vi "Resistance Test_ver2_2.vi"(0 "DMM ref in":refnum<visa-resource-name>, 1 "Measure\nMax Voltage":dbl=100.0, 2 "Resistance Test REF":refnum<vi>, 3 "Resistance Test Stop REF":refnum<vi>, 5 "DMM error in":errorcluster, 7 "Channel  Count":i32, 9 "ESP32 ref in":refnum<visa-resource-name>="COM4", 11 "ESP32 error in":errorcluster, 12 "Wait Current Stable Period":u32, 13 "Manual Trigger Delay (1 s)":dbl=1.0, 14 "Current Sense \nResitance Array":dbl[](array[numeric])) -> (10 "ESP32 ref out":refnum<visa-resource-name>, 15 "ESP32 error out":errorcluster)   [LabVIEW 2023]
uses:
  <instrlib>/Agilent 3446X Series/Agilent 3446X Series.lvlib
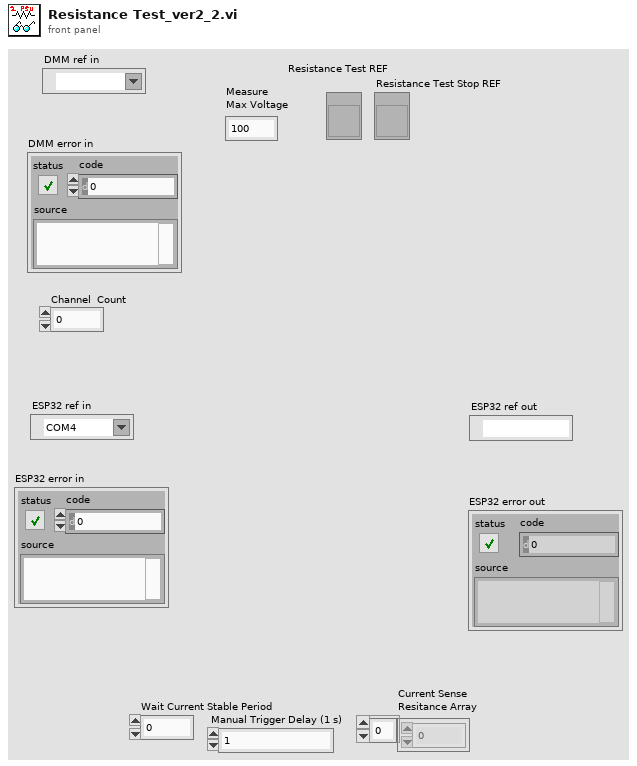
[diagram p1: front panel]
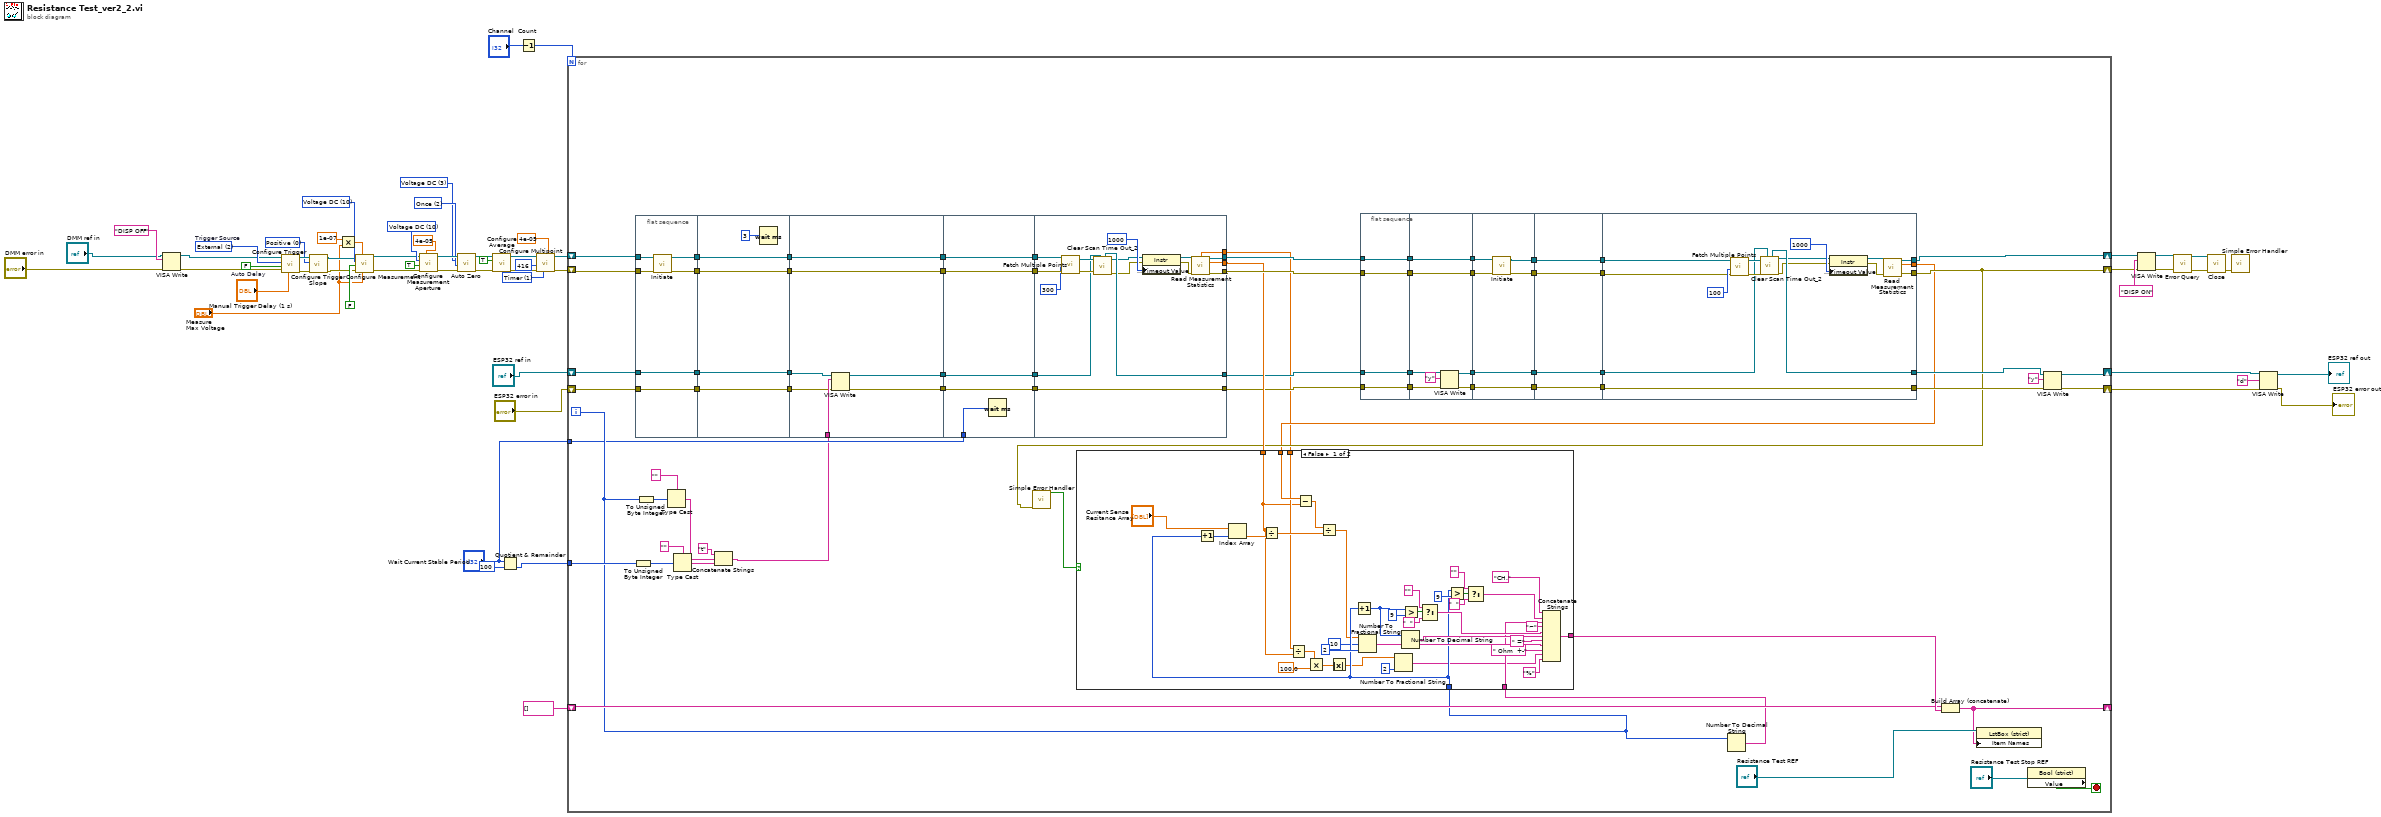
[diagram p0: block diagram]
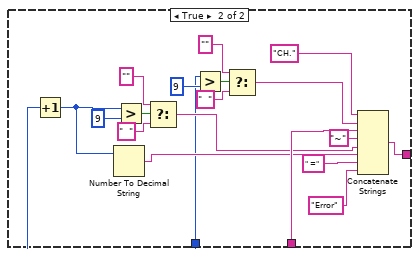
[diagram p2: hidden frame]
diagram:
  w19 = 0 items=["Positive", "Negative"] ("Trigger Edge (1: Negative)")
  w17 = 2 items=["Immediate", "Software (Bus)", "External"]  # Trigger Source
  w18 = FALSE  # Auto Delay
  w25 = 10 items=["Continuity", "Current AC", "Current DC", "Diode", "Frequency", "Resistance 4-wire", "Period", "Resistance 2-wire", "Temperature", "Voltage AC", "Voltage DC", "Voltage DC Ratio", "Capacitance"] ("Measurement Function (10: Voltage DC)")
  w29 = 1 items=["Immediate", "Timer"] ("Sample Source (0: Immediate)")
  w36 = 3 items=["Current DC", "Resistance", "Temperature", "Voltage DC"] ("Zero Type (0: Current DC)")
  w37 = 2 items=["Disable", "Enable", "Once"] ("Auto Zero (1: Enable)")
  w33 = 10 items=["Continuity", "Current AC", "Current DC", "Diode", "Frequency", "Resistance 4-wire", "Period", "Resistance 2-wire", "Temperature", "Voltage AC", "Voltage DC", "Voltage DC Ratio", "Capacitance"] ("Measurement Function (0: Continuity)")
  n1 = VISA Write(VISA resource name="DMM ref in", write buffer="DISP OFF", error in (no error)="DMM error in") -> (VISA resource name out=w4:refnum<visa-resource-name>, error out=w3:errorcluster)  [unwired: 1 out]
  n2 = call <instrlib>:"Configure Trigger.vi"("Manual Trigger Delay (1 s)"="Manual Trigger Delay (1 s)", "error in (no error)"=w3, "Auto Delay (F:Disable)"=w18, "Trigger Source (0: Immediate)"=w17, "VISA resource name"=w4) -> ("error out"=w21:errorcluster, "VISA resource name out"=w20:refnum<visa-resource-name>)  [unwired: 1 in, 4 out]
  n3 = call <instrlib>:"Configure Trigger Slope.vi"("error in (no error)"=w21, "Trigger Edge (1: Negative)"=w19, "VISA resource name"=w20) -> ("error out"=w15:errorcluster, "VISA resource name out"=w16:refnum<visa-resource-name>)  [unwired: 7 in]
  n4 = Multiply(x=1e-07, y="Measure\nMax Voltage") -> (x*y=w26:dbl)
  n5 = call <instrlib>:"Configure Measurement.vi"("Manual Range (1)"="Measure\nMax Voltage", "Absolute Resolution (1E-6)"=w26, "error in (no error)"=w15, "Auto Range (T: Enable)"=FALSE, "Measurement Function (10: Voltage DC)"=w25, "VISA resource name"=w16) -> ("error out"=w22:errorcluster, "VISA resource name out"=w23:refnum<visa-resource-name>)  [unwired: 4 out]
  n6 = call <instrlib>:"Configure Measurement Aperture.vi"("Aperture Time (0.1s)"=4e-05, "error in (no error)"=w22, "Enable Aperture (F: Disable)"=TRUE, "Measurement Function (0: Continuity)"=w33, "VISA resource name"=w23) -> ("error out"=w40:errorcluster, "VISA resource name out"=w39:refnum<visa-resource-name>)  [unwired: 5 in]
  n7 = call <instrlib>:"Auto Zero.vi"("error in (no error)"=w40, "Auto Zero (1: Enable)"=w37, "Zero Type (0: Current DC)"=w36, "VISA resource name"=w39) -> ("error out"=w42:errorcluster, "VISA resource name out"=w41:refnum<visa-resource-name>)  [unwired: 6 in]
  n8 = call <instrlib>:"Configure Average.vi"("error in (no error)"=w42, "Enable Statistics (F: Disable)"=TRUE, "VISA resource name"=w41) -> ("error out"=w31:errorcluster, "VISA resource name out"=w32:refnum<visa-resource-name>)  [unwired: 7 in]
  n9 = Quotient & Remainder(x="Wait Current Stable Period", y=100) -> (floor(x/y)=w11:u32)  [unwired: 1 out]
  n10 = Decrement(x="Channel  Count") -> (x-1=w9:i32)
  n11 = call <instrlib>:"Configure Multipoint.vi"("Sample Interval (1 Second)"=4e-05, "Sample Source (0: Immediate)"=w29, "error in (no error)"=w31, "Sample Count (1)"=416, "VISA resource name"=w32) -> ("error out"=w13:errorcluster, "VISA resource name out"=w14:refnum<visa-resource-name>)  [unwired: 2 in, 3 out]
  n12 = for {
    N: w9 -> [_]
    shift-right: [w82] -> w44
    shift-left: "ESP32 ref in" -> [w111]
    shift-right: [w80] -> w10
    shift-left: "ESP32 error in" -> [w109]
    shift-right: [w78] -> w45
    shift-left: w13 -> [w115]
    shift-right: [w121] -> w46
    shift-left: w14 -> [w116]
    shift-right: [w122] -> _
    shift-left: string[] [] -> [w124]
    tunnel: w11 -> [w99]
    tunnel: "Wait Current Stable Period" -> [w86]
    i -> [w97]
    stop <- w126 stop-if-true
    n13 = To Unsigned Byte Integer(number=w99) -> (unsigned 8bit integer=w103:u8)
    n14 = flat-sequence {
      tunnel: w115 -> [w225]
      tunnel: w116 -> [w227]
      tunnel: [w226] -> w120
      tunnel: [w224] -> w119
      tunnel: [w223] -> w112
      tunnel: w111 -> [w223]
      tunnel: w109 -> [w222]
      tunnel: [w222] -> w108
      tunnel: [w232] -> w118
      tunnel: [w231] -> w117
      tunnel: w120 -> [w232]
      tunnel: w119 -> [w231]
      tunnel: w112 -> [w229]
      tunnel: [w229] -> w110
      tunnel: w108 -> [w228]
      tunnel: [w228] -> w107
      tunnel: w118 -> [w239]
      tunnel: [w239] -> w92
      tunnel: w117 -> [w238]
      tunnel: [w238] -> w94
      tunnel: w110 -> [w237]
      tunnel: w107 -> [w235]
      tunnel: w79 -> [w236]
      tunnel: [w234] -> w90
      tunnel: [w233] -> w88
      tunnel: w94 -> [w244]
      tunnel: [w244] -> w93
      tunnel: w92 -> [w243]
      tunnel: [w243] -> w91
      tunnel: w90 -> [w242]
      tunnel: [w242] -> w89
      tunnel: w88 -> [w241]
      tunnel: [w241] -> w87
      tunnel: w86 -> [w240]
      tunnel: [w258] -> w113
      tunnel: [w259] -> w114
      tunnel: w93 -> [w261]
      tunnel: w91 -> [w260]
      tunnel: [w251] -> w95
      tunnel: w89 -> [w252]
      tunnel: [w256] -> w85
      tunnel: w87 -> [w256]
      tunnel: [w255] -> w96
      tunnel: [w245] -> w59
      frame #0 {
        n15 = call <instrlib>:"Initiate.vi"("error in (no error)"=w225, "VISA resource name"=w227) -> ("error out"=w224:errorcluster, "VISA resource name out"=w226:refnum<visa-resource-name>)  [unwired: 8 out]
      }
      frame #1 {
        n16 = Wait (ms)(milliseconds to wait=u32 3) -> ()  [unwired: 1 out]
      }
      frame #2 {
        n17 = VISA Write(VISA resource name=w237, write buffer=w236, error in (no error)=w235) -> (VISA resource name out=w234:refnum<visa-resource-name>, error out=w233:errorcluster)  [unwired: 1 out]
      }
      frame #3 {
        n18 = Wait (ms)(milliseconds to wait=w240) -> ()  [unwired: 1 out]
      }
      frame #4 {
        n19 = call <instrlib>:"Fetch Multiple Points.vi"("error in (no error)"=w261, "Timeout (10000 ms)"=300, "VISA resource name"=w260) -> ("error out"=w253:errorcluster, "VISA resource name out"=w254:refnum<visa-resource-name>)  [unwired: 1 in, 6 out]
        n20 = call "Clear Scan Time Out_2.vi"("ESP32 ref"=w252, "error in (no error)"=w253, "VISA Refnum in"=w254) -> ("error out"=w248:errorcluster, "VISA Refnum out"=w249:refnum<visa-resource-name>, "ESP32 ref out"=w251:refnum<visa-resource-name>)  [unwired: 4 in, 2 out]
        n21 = property class="Instr"(reference=w249, error in=w248, "General Settings:Timeout Value"=u32 1000) -> (reference out=w247:refnum<visa-resource-name>, error out=w246:errorcluster)
        n22 = call <instrlib>:"Read Measurement Statistics.vi"("VISA resource name"=w247, "error in (no error)"=w246) -> ("Standard Deviation"=w245:dbl, "VISA resource name out"=w259:refnum<visa-resource-name>, "Arithmetic Mean"=w255:dbl, "error out"=w258:errorcluster)  [unwired: 6 in, 4 out]
      }
    }
    n23 = To Unsigned Byte Integer(number=w97) -> (unsigned 8bit integer=w100:u8)
    n24 = Type Cast(type="" ("string"), x=w100) -> (*(type *) &x=w101:string)
    n25 = Type Cast(type="" ("string"), x=w103) -> (*(type *) &x=w102:string)
    n26 = Concatenate Strings("t" ("data in"), w101, w102) -> (w79:string)
    n27 = call <vilib>:"Simple Error Handler.vi"("error in (no error)"=w78) -> ("error?"=w77:bool)  [unwired: 4 in, 4 out]
    n28 = flat-sequence {
      tunnel: w85 -> [w128]
      tunnel: w95 -> [w129]
      tunnel: w113 -> [w130]
      tunnel: w114 -> [w131]
      tunnel: [w131] -> w76
      tunnel: [w130] -> w75
      tunnel: [w129] -> w74
      tunnel: [w128] -> w73
      tunnel: [w138] -> w72
      tunnel: [w137] -> w71
      tunnel: [w135] -> w70
      tunnel: [w132] -> w69
      tunnel: w76 -> [w138]
      tunnel: w75 -> [w137]
      tunnel: w74 -> [w136]
      tunnel: w73 -> [w133]
      tunnel: w72 -> [w142]
      tunnel: w71 -> [w141]
      tunnel: [w140] -> w68
      tunnel: w70 -> [w144]
      tunnel: [w144] -> w67
      tunnel: w69 -> [w143]
      tunnel: [w143] -> w66
      tunnel: [w139] -> w65
      tunnel: w68 -> [w148]
      tunnel: [w148] -> w64
      tunnel: w67 -> [w147]
      tunnel: [w147] -> w63
      tunnel: w66 -> [w146]
      tunnel: [w146] -> w62
      tunnel: w65 -> [w145]
      tunnel: [w145] -> w61
      tunnel: [w164] -> w60
      tunnel: [w162] -> w121
      tunnel: [w161] -> w78
      tunnel: [w157] -> w83
      tunnel: w64 -> [w149]
      tunnel: w63 -> [w158]
      tunnel: w62 -> [w151]
      tunnel: [w151] -> w81
      tunnel: w61 -> [w150]
      frame #0 {
      }
      frame #1 {
        n29 = VISA Write(VISA resource name=w136, write buffer="y", error in (no error)=w133) -> (VISA resource name out=w135:refnum<visa-resource-name>, error out=w132:errorcluster)  [unwired: 1 out]
      }
      frame #2 {
        n30 = call <instrlib>:"Initiate.vi"("error in (no error)"=w141, "VISA resource name"=w142) -> ("error out"=w140:errorcluster, "VISA resource name out"=w139:refnum<visa-resource-name>)  [unwired: 8 out]
      }
      frame #3 {
      }
      frame #4 {
        n31 = call <instrlib>:"Fetch Multiple Points.vi"("error in (no error)"=w149, "Timeout (10000 ms)"=100, "VISA resource name"=w150) -> ("error out"=w159:errorcluster, "VISA resource name out"=w160:refnum<visa-resource-name>)  [unwired: 1 in, 6 out]
        n32 = call "Clear Scan Time Out_2.vi"("ESP32 ref"=w158, "error in (no error)"=w159, "VISA Refnum in"=w160) -> ("error out"=w152:errorcluster, "VISA Refnum out"=w153:refnum<visa-resource-name>, "ESP32 ref out"=w157:refnum<visa-resource-name>)  [unwired: 4 in, 2 out]
        n33 = property class="Instr"(reference=w153, error in=w152, "General Settings:Timeout Value"=u32 1000) -> (reference out=w155:refnum<visa-resource-name>, error out=w154:errorcluster)
        n34 = call <instrlib>:"Read Measurement Statistics.vi"("VISA resource name"=w155, "error in (no error)"=w154) -> ("VISA resource name out"=w162:refnum<visa-resource-name>, "Arithmetic Mean"=w164:dbl, "error out"=w161:errorcluster)  [unwired: 6 in, 5 out]
      }
    }
    n35 = Number To Decimal String(number=w97) -> (decimal integer string=w98:string)  [unwired: 1 in]
    n36 = case shown="False" w77 {
      tunnel: [w197 w216] -> w125
      tunnel: w98 -> [w180 w213]
      tunnel: w60 -> [w168 _]
      tunnel: w97 -> [w181 w204]
      tunnel: w96 -> [w165 _]
      tunnel: w59 -> [w166 _]
      frame False {
        n37 = Increment(x=w181) -> (x+1=w185:i32)
        n38 = Index Array(array="Current Sense \nResitance Array", index=w185) -> (element=w179:dbl)
        n39 = Divide(x=w165, y=w179) -> (x/y=w177:dbl)
        n40 = Divide(x=w166, y=w165) -> (x/y=w174:dbl)
        n41 = Subtract(x=w168, y=w165) -> (x-y=w178:dbl)
        n42 = Multiply(x=w174, y=100.0) -> (x*y=w171:dbl)
        n43 = Divide(x=w178, y=w177) -> (x/y=w176:dbl)
        n44 = Absolute Value(x=w171) -> (abs(x)=w167:dbl)
        n45 = Increment(x=w181) -> (x+1=w188:i32)
        n46 = Number To Fractional String(number=w176, width (-)=i16 10, precision (6)=i16 2) -> (F-format string=w183:string)  [unwired: 1 in]
        n47 = Number To Fractional String(number=w167, precision (6)=i16 2) -> (F-format string=w170:string)  [unwired: 2 in]
        n48 = Number To Decimal String(number=w188) -> (decimal integer string=w187:string)  [unwired: 1 in]
        n49 = Greater?(x=w188, y=9) -> (0:w192:bool)
        n50 = Select(t="" ("string"), s=w192, f="  " ("string")) -> (s? t:f=w189:string)
        n51 = Greater?(x=w181, y=9) -> (0:w200:bool)
        n52 = Select(t="" ("string"), s=w200, f="  " ("string")) -> (s? t:f=w195:string)
        n53 = Concatenate Strings("CH." ("string"), w195, w180, "~" ("string"), w189, w187, " =" ("string"), w183, " Ohm  +-" ("string"), w170, "%" ("string")) -> (w197:string)
      }
      frame True {
        n54 = Increment(x=w204) -> (x+1=w206:i32)
        n55 = Number To Decimal String(number=w206) -> (decimal integer string=w205:string)  [unwired: 1 in]
        n56 = Greater?(x=w206, y=9) -> (0:w210:bool)
        n57 = Select(t="" ("string"), s=w210, f="  " ("string")) -> (s? t:f=w207:string)
        n58 = Greater?(x=w204, y=9) -> (0:w219:bool)
        n59 = Select(t="" ("string"), s=w219, f="  " ("string")) -> (s? t:f=w214:string)
        n60 = Concatenate Strings("CH." ("string"), w214, w213, "~" ("string"), w207, w205, " =" ("string"), "Error" ("string")) -> (w216:string)
      }
    }
    n61 = Build Array (concatenate)(w124, w125) -> (w122:string[])
    n62 = property class="LstBox (strict)"(reference="Resistance Test REF", "Item Names"=w122) -> ()  [unwired: 1 in, 2 out]
    n63 = property class="Bool (strict)"(reference="Resistance Test Stop REF") -> ("Value"=w126:bool)  [unwired: 1 in, 2 out]
    n64 = VISA Write(VISA resource name=w83, write buffer="y", error in (no error)=w81) -> (VISA resource name out=w82:refnum<visa-resource-name>, error out=w80:errorcluster)  [unwired: 1 out]
  }
  n65 = VISA Write(VISA resource name=w46, write buffer="DISP ON", error in (no error)=w45) -> (VISA resource name out=w53:refnum<visa-resource-name>, error out=w52:errorcluster)  [unwired: 1 out]
  n66 = call <instrlib>:"Error Query.vi"("error in (no error)"=w52, "VISA resource name"=w53) -> ("error out"=w58:errorcluster, "VISA resource name out"=w57:refnum<visa-resource-name>)  [unwired: 8 out]
  n67 = call <instrlib>:"Close.vi"("error in (no error)"=w58, "VISA resource name"=w57) -> ("error out"=w56:errorcluster)  [unwired: 9 out]
  n68 = call <vilib>:"Simple Error Handler.vi"("error in (no error)"=w56) -> ()  [unwired: 1 in, 8 out]
  n69 = VISA Write(VISA resource name=w44, write buffer="d" ("data in"), error in (no error)=w10) -> (VISA resource name out=→"ESP32 ref out":refnum<visa-resource-name>, error out=→"ESP32 error out":errorcluster)  [unwired: 1 out]
